vi "读取有多少张表单.vi"(8 "错误输入（无错误）":errorcluster, 11 "所有表单引用":refnum<k7>) -> (0 "错误输出":errorcluster, 2 "表单个数":i32, 3 "所有表单引用输出":refnum<k7>)   [LabVIEW 2013, in "excel处理.lvlib"]
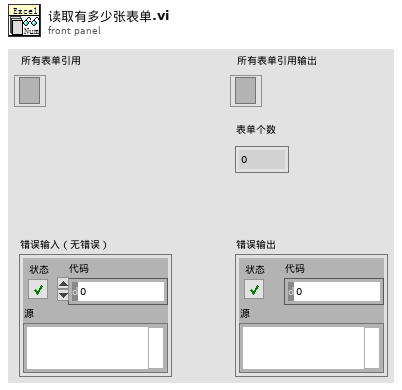
[diagram p1: front panel]
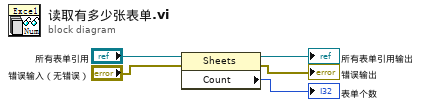
[diagram p0: block diagram]
diagram:
  n1 = property on="属性节点" class="Sheets"(reference="所有表单引用", error in="错误输入（无错误）") -> (reference out=→"所有表单引用输出":refnum<k7>, error out=→"错误输出":errorcluster, "Count"=→"表单个数":i32)
